vi "Write Chars To File.vi"(0 "convert eol? (no:F)":bool, 1 "display dialog? (F)":bool, 3 "append to file? (new file:F)":bool, 4 "character string":string, 5 "file path (dialog if empty)":path) -> (2 "new file path (Not A Path if cancelled)":path)   [LabVIEW 2013]
doc: "This is a modified version of the \"Write Characters to File.vi\" found in the file I/O toolbox. This version will not prompt the user when replacing an existing file unless the new input \"display dialog? (F)\" is set TRUE. AutoCon, 2/98\n\nWrites a character string to a new byte stream file or appends the string to an existing file. The VI opens or creates the file beforehand and closes it afterwards.\n\nfile path is the path name of the file. If file path is empty (default value) or is Not A Path, the VI displays a File dialog box from which you can select a file. Error 43 occurs if the user cancels the dialog. \n\ncharacter string is the data the VI writes to the file.\n\nappend to file? Set to TRUE if you want to append the data to a existing file; you can also set it TRUE to write to a new file. Set to FALSE (default value) if you want to write the data to a new file or to replace an existing file.\n\nnew file path is the path of the file to which the VI wrote data. You can use this output to determine the path of a file that you open using dialog. new file path returns Not A Path if the user selects Cancel from the dialog box."
panel:
  # "Modified to prevent replacement dialog - AutoCon 11/97"
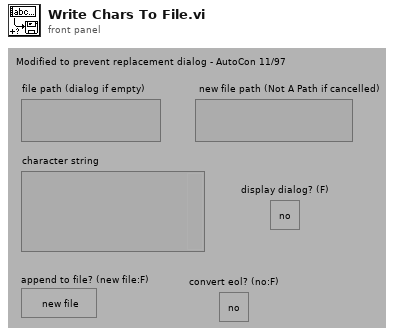
[diagram p1: front panel]
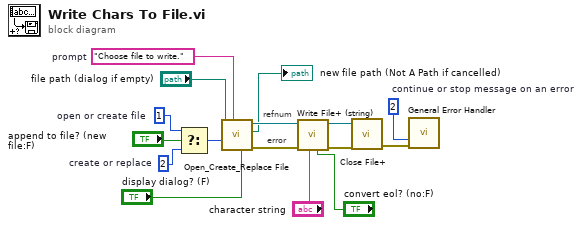
[diagram p0: block diagram]
diagram:
  w5 = i16 2  # create or replace
  w14 = 2  # continue or stop message on an error
  w11 = "Choose file to write."  # prompt
  w8 = i16 1  # open or create file
  # "error"
  # "refnum"
  n1 = Select(t=w8, s="append to file? (new file:F)", f=w5) -> (s? t:f=w10:i16)
  n2 = call <vilib>:"Open_Create_Replace File.vi"("advisory dialog? (display:T)"="display dialog? (F)", "prompt"=w11, "function (open:0)"=w10, "file path"="file path (dialog if empty)") -> ("error out"=w15:errorcluster, "new file path"=→"new file path (Not A Path if cancelled)":path, "refnum"=w4:refnum<file>)  [unwired: 4 in, 1 out]
  n3 = call <vilib>:"Write File+ (string).vi"("convert eol? (no:F)"="convert eol? (no:F)", "string"="character string", "error in (no error)"=w15, "refnum"=w4) -> ("error out"=w13:errorcluster, "dup refnum"=w12:refnum<file>)  [unwired: 3 in, 1 out]
  n4 = call <vilib>:"Close File+.vi"("error in (no error)"=w13, "refnum"=w12) -> ("error out"=w9:errorcluster)  [unwired: 3 in, 2 out]
  n5 = call <vilib>:"General Error Handler.vi"("type of dialog (OK msg:1)"=w14, "error in (no error)"=w9) -> ()  [unwired: 9 in, 5 out]
